vi "read_H.vi"(8 "error in (no error)":errorcluster, 11 "NMF in":refnum<class "NMF.lvclass">) -> (0 "error out":errorcluster, 2 "H":dbl[][](array[numeric]), 3 "NMF out":refnum<class "NMF.lvclass">)   [LabVIEW 2020, in "NMF.lvclass"]
uses:
  NMF.lvclass
  NMF.lvclass/NMF.ctl
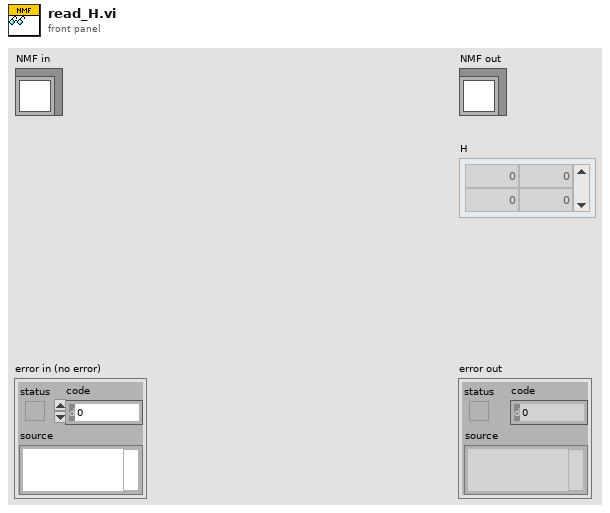
[diagram p1: front panel]
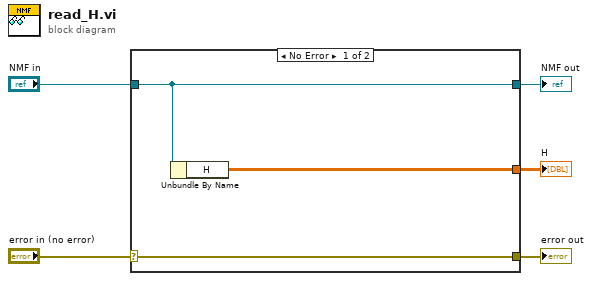
[diagram p0: block diagram]
diagram:
  n1 = case shown="No Error" "error in (no error)" {
    selector: "error in (no error)" -> [w8 w9]
    tunnel: [w8 w9] -> w4
    tunnel: [w7 w10] -> w2
    tunnel: "NMF in" -> [w7 w10]
    tunnel: [w6 _] -> w1
    frame No Error {
      n2 = Unbundle By Name(w7) -> ("H"=w6:dbl[][])
    }
    frame Error {
    }
  }
  "error out" <- w4
  "NMF out" <- w2
  "H" <- w1
